vi "SeqBuilder.vi"(7 "Config Cluster":T1, 8 "error in":errorcluster, 9 "Script name":string, 10 "Engine Ref out":refnum<k7>, 11 "TestStand UI Application Manager (out)":refnum<k7>) -> (0 "error out":errorcluster)   [LabVIEW 2010]
uses:
  Config cluster.ctl
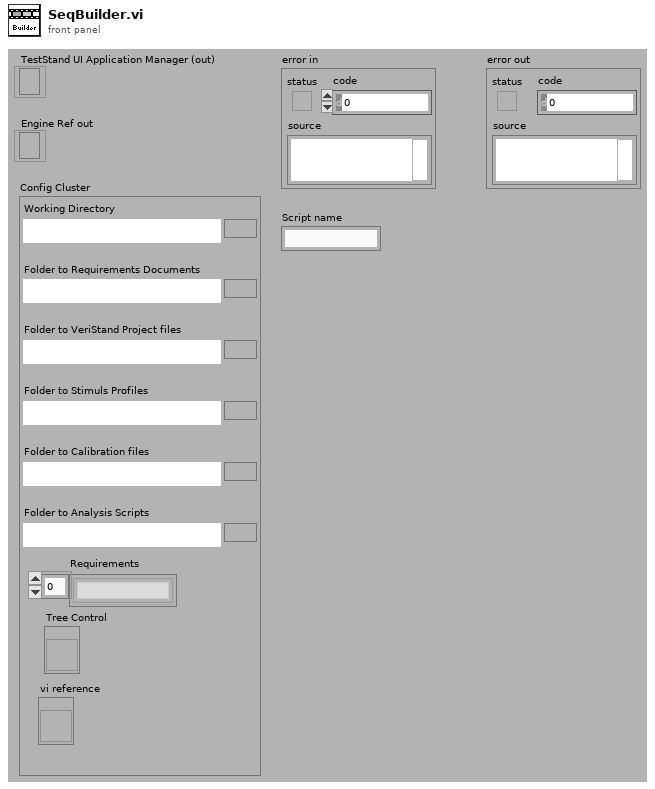
[diagram p1: front panel]
types:
  T1 = typedef "Config cluster.ctl" = cluster{"Working Directory":path, "Folder to Requirements Documents":path, "Folder to VeriStand Project files":path, "Folder to Stimuls Profiles":path, "Folder to Calibration files":path, "Folder to Analysis Scripts":path, "Requirements":string[], "Tree Control":refnum<vi>, "vi reference":refnum<vi>}
  T2 = typedef "SeqStepTypeDef.ctl" = cluster{"Step Type":T3, "Tag":string, "Step component":string, "Req":string, "Symbol Index":i32, "Conditional":bool, "Attended?":bool, "Paths":T4, "Indent Level":i32}
  T3 = typedef "TestComponents.ctl" = enum16{"Script", "Test Procedure", "VS_Project", "Calibration File", "Stimulus Profile", "Analysis Script"}
  T4 = typedef "FilePaths.ctl" = cluster{"Project Files  Path":string, "Calibration Files Path":string, "Stimulus Files Path":string, "Analysis File path":string, "Working Directory":string}
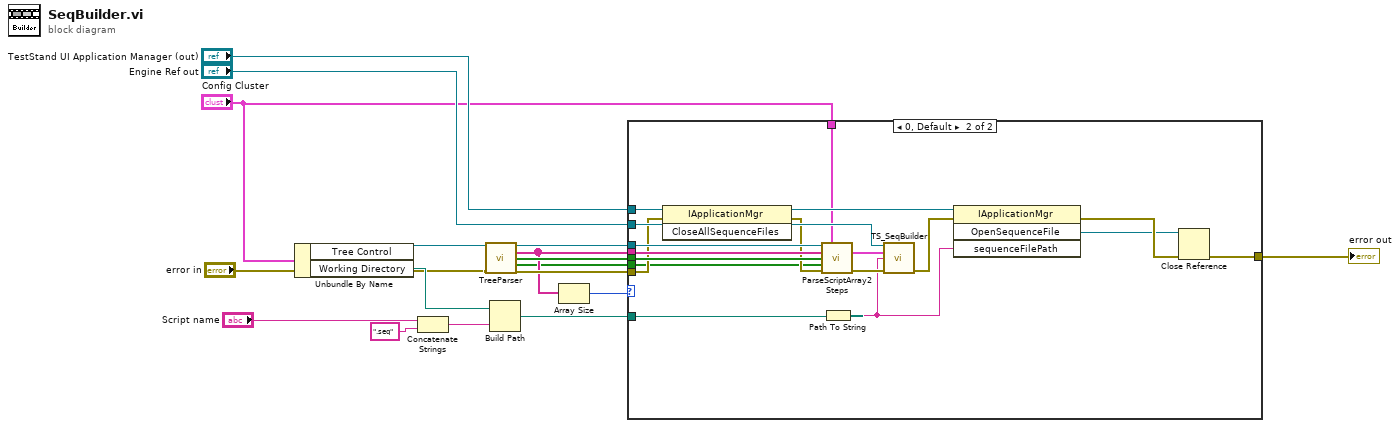
[diagram p0: block diagram]
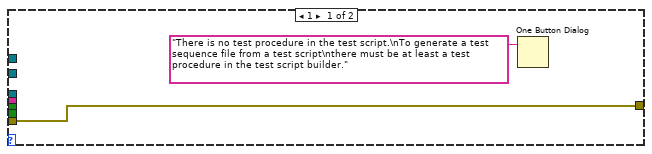
[diagram p2: hidden frame]
diagram:
  n1 = Unbundle By Name("Config Cluster") -> ("Tree Control"=w6:refnum<vi>, "Working Directory"=w12:path)
  n2 = Concatenate Strings("Script name", ".seq" ("string")) -> (w14:string)
  n3 = call "TreeParser.vi"("Tree ref in"=w6, "error in (no error)"="error in") -> ("Tree Ref out"=w7:refnum<vi>, "Script Array"=w8:string[], "Conditional Array out"=w15:bool[], "Attended? Array"=w2:bool[], "error out"=w11:errorcluster)  [unwired: 9 in]
  n4 = Build Path(base path=w12, name or relative path=w14) -> (appended path=w13:path)
  n5 = Array Size(array=w8) -> (size(s)=w9:i32)
  n6 = case shown="0, Default" w9 {
    tunnel: w11 -> [w19 w26]
    tunnel: w7 -> [_ w37]
    tunnel: [w19 w36] -> w17
    tunnel: "TestStand UI Application Manager (out)" -> [_ w35]
    tunnel: w8 -> [_ w33]
    tunnel: w13 -> [_ w31]
    tunnel: w15 -> [_ w29]
    tunnel: "Engine Ref out" -> [_ w28]
    tunnel: w2 -> [_ w21]
    tunnel: "Config Cluster" -> [_ w20]
    frame 1 {
      n7 = One Button Dialog(message="There is no test procedure in the test script.\nTo generate a test sequence file from a test script\nthere must be at least a test procedure in the test script builder.") -> ()  [unwired: 1 in, 1 out]
    }
    frame 0, Default {
      n8 = invoke class="IApplicationMgr" method="CloseAllSequenceFiles"(reference=w35, error in=w26) -> (reference out=w27:refnum<k7>, error out=w25:errorcluster)  [unwired: 1 in, 1 out]
      n9 = call "ParseScriptArray2Steps.vi"("Tree Ref in"=w37, "Config Cluster out"=w20, "Script Array"=w33, "Conditional Array out"=w29, "Attended? Array"=w21, "error in"=w25) -> ("Steps with Params"=w32:T2[], "error out"=w30:errorcluster)  [unwired: 7 in, 1 out]
      n10 = Path To String(path=w31) -> (string=w22:string)
      n11 = call "TS_SeqBuilder.vi"("Engine Ref"=w28, "Steps array"=w32, "Test Sequence File (Save As)"=w22, "error in"=w30) -> ("error out"=w34:errorcluster)  [unwired: 11 in]
      n12 = invoke class="IApplicationMgr" method="OpenSequenceFile"(reference=w27, error in=w34, "sequenceFilePath"=w22) -> (error out=w24:errorcluster, "OpenSequenceFile"=w23:refnum<k7>)  [unwired: 1 in, 2 out]
      n13 = Close Reference(reference=w23, error in (no error)=w24) -> (error out=w36:errorcluster)
    }
  }
  "error out" <- w17
